vi "ipconfig.vi"   [LabVIEW 2012]
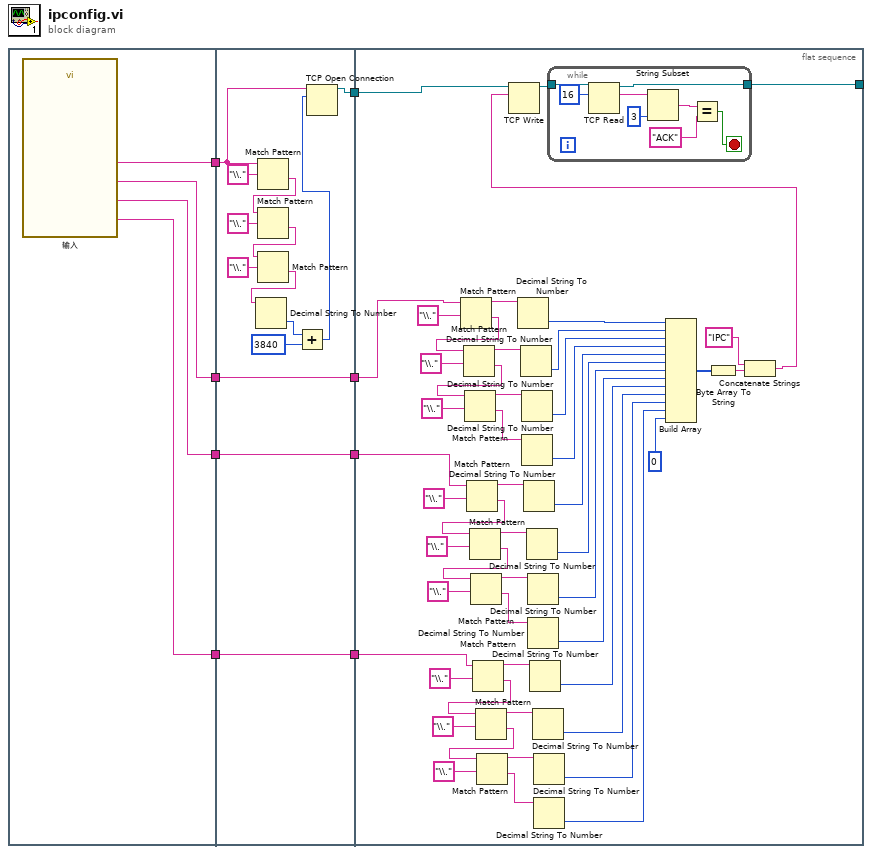
[diagram p0: block diagram]
diagram:
  n1 = flat-sequence {
    tunnel: [w12] -> w4
    tunnel: [w11] -> w3
    tunnel: [w10] -> w2
    tunnel: [w9] -> w1
    tunnel: [w26] -> w8
    tunnel: w4 -> [w20]
    tunnel: [w16] -> w7
    tunnel: w3 -> [w16]
    tunnel: [w15] -> w6
    tunnel: w2 -> [w15]
    tunnel: [w14] -> w5
    tunnel: w1 -> [w14]
    tunnel: w8 -> [w76]
    tunnel: w7 -> [w29]
    tunnel: w6 -> [w28]
    tunnel: w5 -> [w27]
    tunnel: [w74] -> _
    frame #0 {
      n2 = call "输入"() -> ("修改网关"=w9:string, "修改子网掩码"=w10:string, "修改IP地址"=w11:string, "原始IP地址"=w12:string)  [unwired: 14 in, 2 out]
    }
    frame #1 {
      n3 = Match Pattern(string=w20, regular expression="\\." ("正则表达式")) -> (after substring=w22:string)  [unwired: 1 in, 3 out]
      n4 = Match Pattern(string=w22, regular expression="\\." ("正则表达式")) -> (after substring=w21:string)  [unwired: 1 in, 3 out]
      n5 = Match Pattern(string=w21, regular expression="\\." ("正则表达式")) -> (after substring=w19:string)  [unwired: 1 in, 3 out]
      n6 = Decimal String To Number(string=w19) -> (number=w18:i32)  [unwired: 2 in, 1 out]
      n7 = Add(x=w18, y=3840) -> (x+y=w13:i32)
      n8 = TCP Open Connection(address=w20, remote port or service name=w13) -> (connection ID=w26:refnum<k5>)  [unwired: 3 in, 1 out]
    }
    frame #2 {
      n9 = Match Pattern(string=w29, regular expression="\\.") -> (before substring=w72:string, after substring=w67:string)  [unwired: 1 in, 2 out]
      n10 = Match Pattern(string=w67, regular expression="\\.") -> (before substring=w70:string, after substring=w66:string)  [unwired: 1 in, 2 out]
      n11 = Match Pattern(string=w66, regular expression="\\.") -> (before substring=w68:string, after substring=w61:string)  [unwired: 1 in, 2 out]
      n12 = Match Pattern(string=w28, regular expression="\\.") -> (before substring=w59:string, after substring=w54:string)  [unwired: 1 in, 2 out]
      n13 = Match Pattern(string=w54, regular expression="\\.") -> (before substring=w57:string, after substring=w53:string)  [unwired: 1 in, 2 out]
      n14 = Match Pattern(string=w53, regular expression="\\.") -> (before substring=w55:string, after substring=w52:string)  [unwired: 1 in, 2 out]
      n15 = Match Pattern(string=w27, regular expression="\\.") -> (before substring=w50:string, after substring=w45:string)  [unwired: 1 in, 2 out]
      n16 = Match Pattern(string=w45, regular expression="\\.") -> (before substring=w48:string, after substring=w44:string)  [unwired: 1 in, 2 out]
      n17 = Match Pattern(string=w44, regular expression="\\.") -> (before substring=w46:string, after substring=w43:string)  [unwired: 1 in, 2 out]
      n18 = Decimal String To Number(string=w72) -> (number=w65:i32)  [unwired: 2 in, 1 out]
      n19 = Decimal String To Number(string=w70) -> (number=w64:i32)  [unwired: 2 in, 1 out]
      n20 = Decimal String To Number(string=w68) -> (number=w63:i32)  [unwired: 2 in, 1 out]
      n21 = Decimal String To Number(string=w61) -> (number=w62:i32)  [unwired: 2 in, 1 out]
      n22 = Decimal String To Number(string=w59) -> (number=w42:i32)  [unwired: 2 in, 1 out]
      n23 = Decimal String To Number(string=w57) -> (number=w41:i32)  [unwired: 2 in, 1 out]
      n24 = Decimal String To Number(string=w55) -> (number=w40:i32)  [unwired: 2 in, 1 out]
      n25 = Decimal String To Number(string=w52) -> (number=w39:i32)  [unwired: 2 in, 1 out]
      n26 = Decimal String To Number(string=w50) -> (number=w38:i32)  [unwired: 2 in, 1 out]
      n27 = Decimal String To Number(string=w48) -> (number=w37:i32)  [unwired: 2 in, 1 out]
      n28 = Decimal String To Number(string=w46) -> (number=w36:i32)  [unwired: 2 in, 1 out]
      n29 = Decimal String To Number(string=w43) -> (number=w35:i32)  [unwired: 2 in, 1 out]
      n30 = Build Array(w65, w64, w63, w62, w42, w41, w40, w39, w38, w37, w36, w35, 0 ("元素")) -> (w33:i32[])
      n31 = Byte Array To String(unsigned byte array=w33) -> (string=w32:string)
      n32 = Concatenate Strings("IPC" ("数据输入"), w32) -> (w30:string)
      n33 = TCP Write(connection ID=w76, data in=w30) -> (connection ID out=w75:refnum<k5>)  [unwired: 2 in, 2 out]
      n34 = while {
        tunnel: w75 -> [w84]
        tunnel: [w78] -> w74
        stop <- w79 stop-if-true
        n35 = TCP Read(connection ID=w84, bytes to read=16 ("读取的字节")) -> (connection ID out=w78:refnum<k5>, data out=w82:string)  [unwired: 3 in, 1 out]
        n36 = String Subset(string=w82, length (rest)=3 ("偏移量(0)")) -> (substring=w81:string)  [unwired: 1 in]
        n37 = Equal?(x=w81, y="ACK") -> (x = y?=w79:bool)
      }
    }
  }
